vi "Glyph_MouseDown.vi"(6 "Double Click":bool, 8 "error in":errorcluster, 9 "Coords":T5, 10 "CtlRef":refnum<vi>, 11 "Data in":T1={"Class"={"Ants"=refnum, "Layer"=refnum, "Templates"=refnum, "Icon"=refnum, "Glyph"=refnum, "Settings"=refnum, "Tools"=refnum}, "Ref"={"Add Layer"=refnum, "Remove Layer"=refnum, "Line Text"=[], "Body Text Spec"=refnum, "DNL_Font"=refnum, "glyph path str"=refnum, "templates path str"=refnum, "Arrow Up"=refnum, "Arrow Down"=refnum, "IE VI Ref"=refnum, "Glyphs tree"=refnum, "Templates tree"=refnum, "Layer Icon Text"=refnum, "Layer Template"=refnum, "Body Text"=refnum, "Search Templates"=refnum, "TextMarker"=refnum, "Tab Control"=refnum, "Search Glyphs"=refnum, "Line Color"=refnum, "DNL_Glyphs []"=refnum, "Fill Color"=refnum, "Tools"=refnum, "Icon"=refnum, "Preview"=refnum, "Ants"=refnum, "Terminals"=refnum, "menu reference"=refnum, "LayerNames"=[], "GlyphLoadAnimation"=refnum, "TemplateLoadAnimation"=refnum, "refreshGlyphs"=refnum, "refreshTemplates"=refnum}, "Support"={"AntsRect"={"left"=0, "top"=0, "right"=0, "bottom"=0}, "Mouse Move Coords"={"Horizontal"=0, "Vertical"=0}, "Mouse Down Coords"={"Horizontal"=0, "Vertical"=0}, "Temp Coord"={"Horizontal"=0, "Vertical"=0}, "Action"=enum."Default", "Edge Color"=4914962, "Fill Color"=16860, "Mouse Down?"=FALSE, "Draft Mode?"=FALSE, "Temp Icon"=bytes[3102], "CTRL Pressed"=FALSE, "Move Selection?"=FALSE, "AntsRect Orig"={"left"=0, "top"=0, "right"=0, "bottom"=0}, "Text"="", "TM Set?"=FALSE, "Mouse inside icon?"=FALSE, "Tool (old value)"=0, "Pencil Move Color"=0, "Swap Colors?"=FALSE, "Shift pressed?"=FALSE}}) -> (0 "error out":errorcluster, 3 "Data out":T1={"Class"={"Ants"=refnum, "Layer"=refnum, "Templates"=refnum, "Icon"=refnum, "Glyph"=refnum, "Settings"=refnum, "Tools"=refnum}, "Ref"={"Add Layer"=refnum, "Remove Layer"=refnum, "Line Text"=[], "Body Text Spec"=refnum, "DNL_Font"=refnum, "glyph path str"=refnum, "templates path str"=refnum, "Arrow Up"=refnum, "Arrow Down"=refnum, "IE VI Ref"=refnum, "Glyphs tree"=refnum, "Templates tree"=refnum, "Layer Icon Text"=refnum, "Layer Template"=refnum, "Body Text"=refnum, "Search Templates"=refnum, "TextMarker"=refnum, "Tab Control"=refnum, "Search Glyphs"=refnum, "Line Color"=refnum, "DNL_Glyphs []"=refnum, "Fill Color"=refnum, "Tools"=refnum, "Icon"=refnum, "Preview"=refnum, "Ants"=refnum, "Terminals"=refnum, "menu reference"=refnum, "LayerNames"=[], "GlyphLoadAnimation"=refnum, "TemplateLoadAnimation"=refnum, "refreshGlyphs"=refnum, "refreshTemplates"=refnum}, "Support"={"AntsRect"={"left"=0, "top"=0, "right"=0, "bottom"=0}, "Mouse Move Coords"={"Horizontal"=0, "Vertical"=0}, "Mouse Down Coords"={"Horizontal"=0, "Vertical"=0}, "Temp Coord"={"Horizontal"=0, "Vertical"=0}, "Action"=enum."Default", "Edge Color"=4914962, "Fill Color"=16860, "Mouse Down?"=FALSE, "Draft Mode?"=FALSE, "Temp Icon"=bytes[3102], "CTRL Pressed"=FALSE, "Move Selection?"=FALSE, "AntsRect Orig"={"left"=0, "top"=0, "right"=0, "bottom"=0}, "Text"="", "TM Set?"=FALSE, "Mouse inside icon?"=FALSE, "Tool (old value)"=0, "Pencil Move Color"=0, "Swap Colors?"=FALSE, "Shift pressed?"=FALSE}})   [LabVIEW 2025]
doc: "Performs the actions necessary when there is a Mouse Down event on the Glyph array."
uses:
  <vilib>/Utility/miscctls.llb/LVPoint32TypeDef.ctl
  <resource>/plugins/NIIconEditor/Controls/Global Data.ctl
  <resource>/plugins/NIIconEditor/Class/Ants/Ants.lvclass
  <resource>/plugins/NIIconEditor/Class/FakedArray/FakedArray.lvclass
  <vilib>/LabVIEW Icon API/lv_icon/Classes/Icon/Icon.lvclass
  <resource>/plugins/NIIconEditor/Class/Icon Library/Glyph.lvclass
  <resource>/plugins/NIIconEditor/Class/Settings/Settings.lvclass
  <resource>/plugins/NIIconEditor/Class/Tools/Tools Paint.lvclass
  <resource>/plugins/NIIconEditor/Controls/IE Classes.ctl
  <resource>/plugins/NIIconEditor/Controls/References Cluster.ctl
  <resource>/plugins/NIIconEditor/Controls/SupportClass.ctl
  <resource>/plugins/NIIconEditor/Controls/SupportClass_Action.ctl
  <vilib>/LabVIEW Icon API/lv_icon/Controls/IEColor.ctl
  <vilib>/LabVIEW Icon API/lv_icon/Controls/Graphic.ctl
  <resource>/plugins/NIIconEditor/Controls/Tools.ctl
  <vilib>/LabVIEW Icon API/lv_icon/lv_icon.lvlib
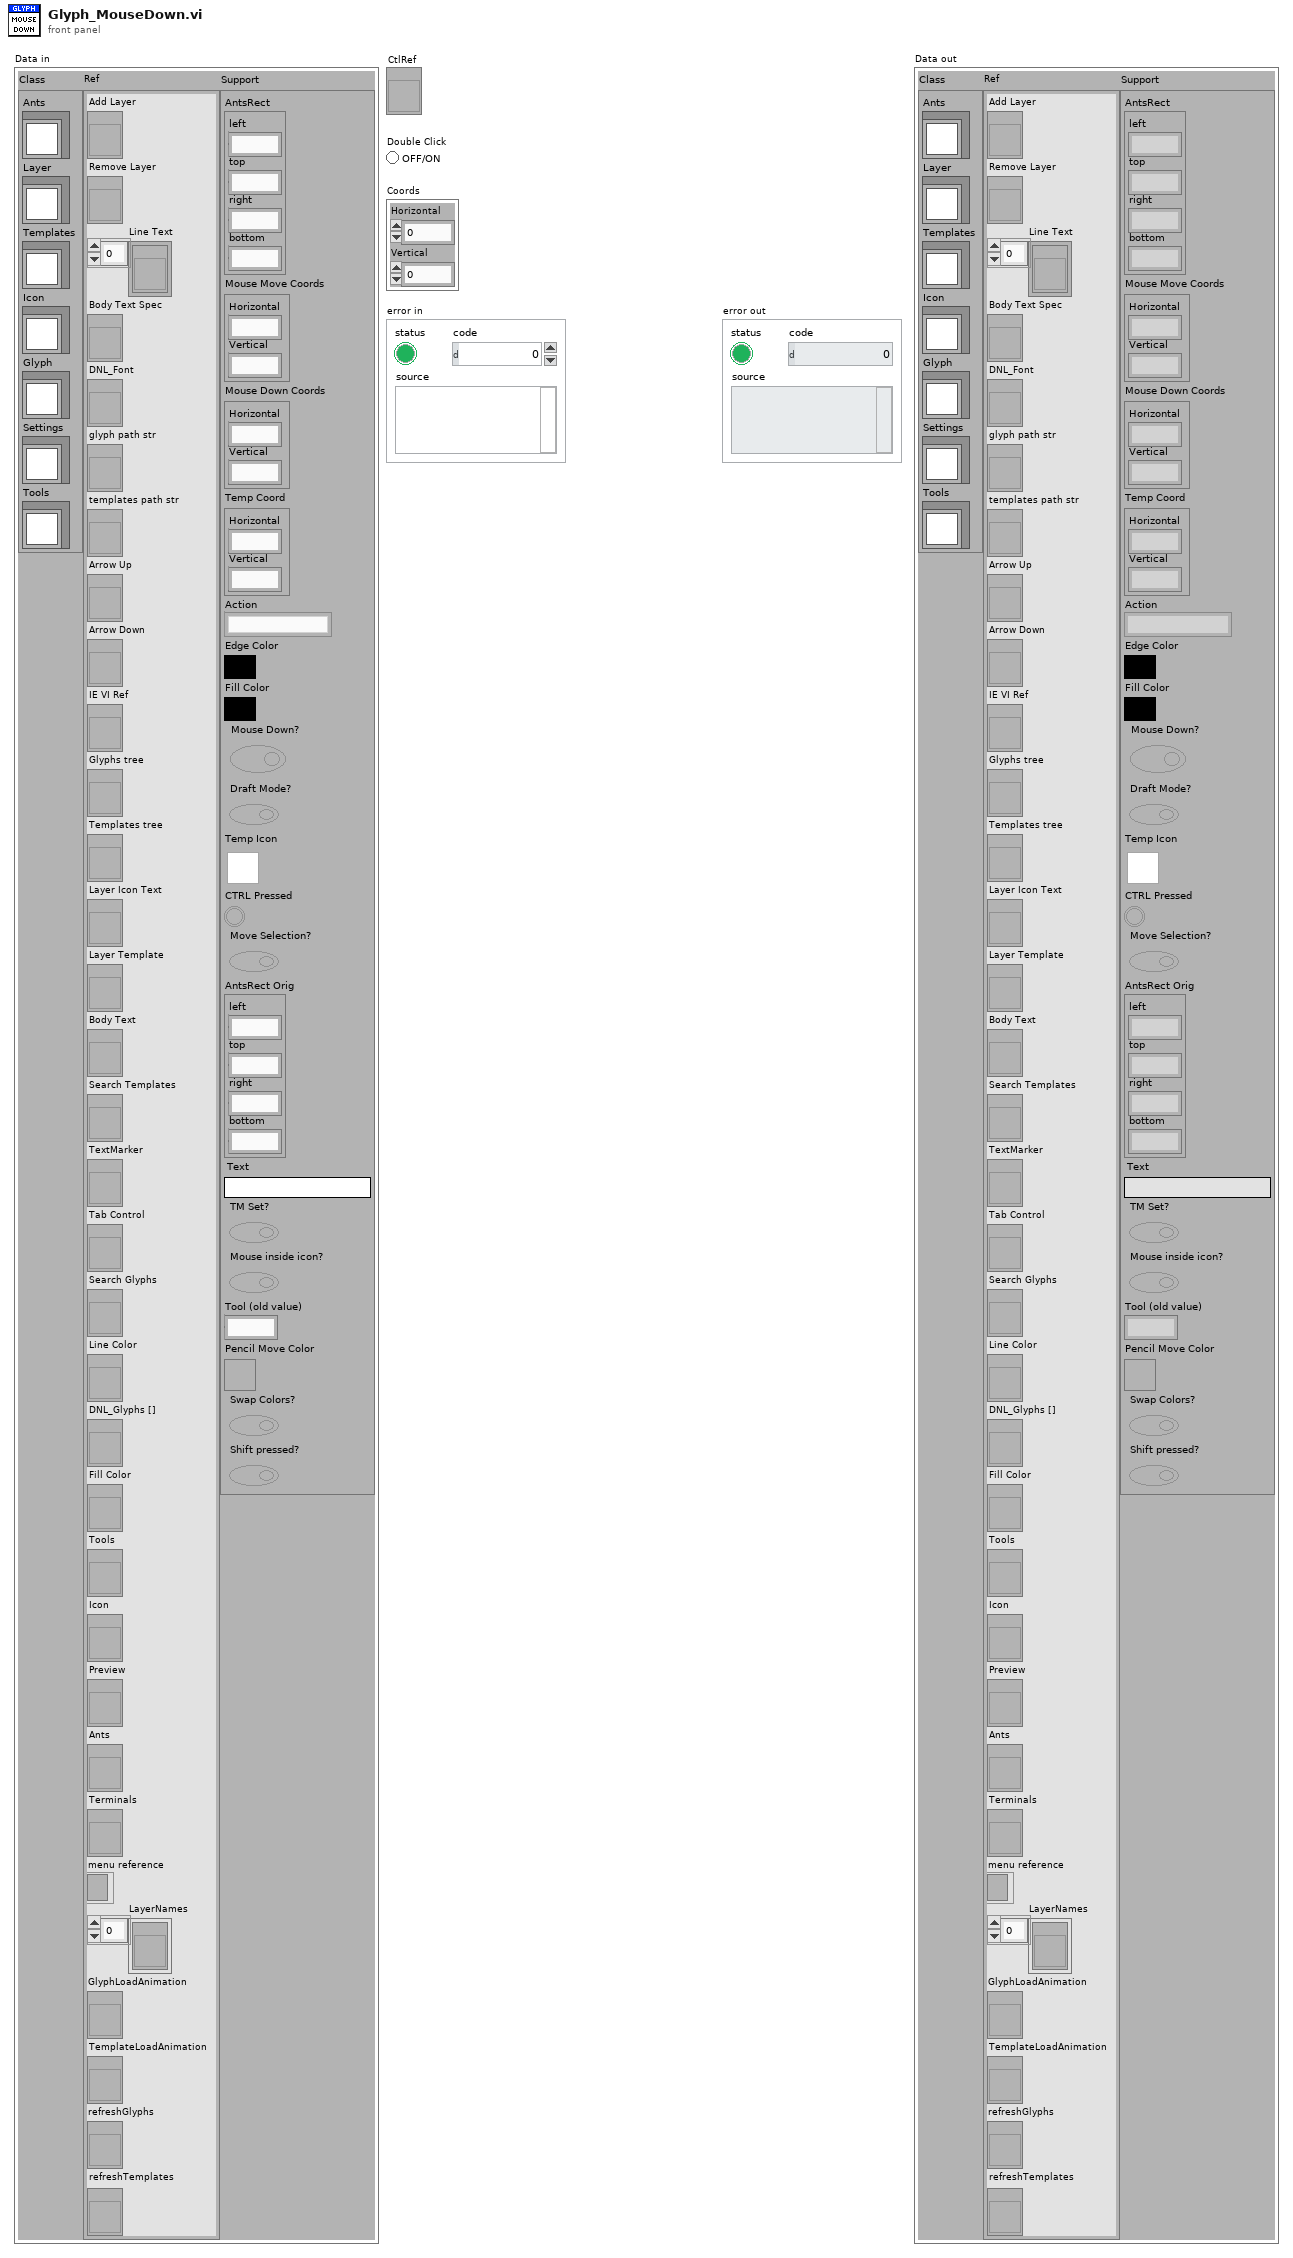
[diagram p1: front panel]
types:
  T1 = typedef "lv_icon.lvlib/Global Data.ctl" = cluster{"Class":T2, "Ref":T3, "Support":T4}
  T2 = typedef "IE Classes.ctl" = cluster{"Ants":refnum<class "Ants.lvclass">, "Layer":refnum<class "FakedArray.lvclass">, "Templates":refnum<class "FakedArray.lvclass">, "Icon":refnum<class "Icon.lvclass">, "Glyph":refnum<class "Glyph.lvclass">, "Settings":refnum<class "Settings.lvclass">, "Tools":refnum<class "Tools Paint.lvclass">}
  T3 = typedef "lv_icon.lvlib/References Cluster.ctl" = cluster{"Add Layer":refnum<vi>, "Remove Layer":refnum<vi>, "Line Text":refnum<vi>[], "Body Text Spec":refnum<vi>, "DNL_Font":refnum<vi>, "glyph path str":refnum<vi>, "templates path str":refnum<vi>, "Arrow Up":refnum<vi>, "Arrow Down":refnum<vi>, "IE VI Ref":refnum<vi>, "Glyphs tree":refnum<vi>, "Templates tree":refnum<vi>, "Layer Icon Text":refnum<vi>, "Layer Template":refnum<vi>, "Body Text":refnum<vi>, "Search Templates":refnum<vi>, "TextMarker":refnum<vi>, "Tab Control":refnum<vi>, "Search Glyphs":refnum<vi>, "Line Color":refnum<vi>, "DNL_Glyphs []":refnum<vi>, "Fill Color":refnum<vi>, "Tools":refnum<vi>, "Icon":refnum<vi>, "Preview":refnum<vi>, "Ants":refnum<vi>, "Terminals":refnum<vi>, "menu reference":refnum<k9>, "LayerNames":refnum<vi>[], "GlyphLoadAnimation":refnum<vi>, "TemplateLoadAnimation":refnum<vi>, "refreshGlyphs":refnum<vi>, "refreshTemplates":refnum<vi>}
  T4 = typedef "SupportClass.ctl" = cluster{"AntsRect":cluster{"left":i16, "top":i16, "right":i16, "bottom":i16}, "Mouse Move Coords":T5, "Mouse Down Coords":T5, "Temp Coord":T5, "Action":T6, "Edge Color":T7, "Fill Color":T7, "Mouse Down?":bool, "Draft Mode?":bool, "Temp Icon":picture, "CTRL Pressed":bool, "Move Selection?":bool, "AntsRect Orig":cluster{"left":i16, "top":i16, "right":i16, "bottom":i16}, "Text":string, "TM Set?":bool, "Mouse inside icon?":bool, "Tool (old value)":u32, "Pencil Move Color":u32, "Swap Colors?":bool, "Shift pressed?":bool}
  T5 = typedef "LVPoint32TypeDef.ctl" = cluster{"Horizontal":i32, "Vertical":i32}
  T6 = typedef "SupportClass_Action.ctl" = enum16{"Default", "Move Selection", "Glyph Library", "Tool"}
  T7 = typedef "IEColor.ctl" = u32
  T8 = typedef "Graphic.ctl" = cluster{"Rectangle":cluster{"left":i16, "top":i16, "right":i16, "bottom":i16}, "Path":path, "Image":picture, "Filter":string, "FileName":string}
  T9 = typedef "Tools.ctl" = enum32{"Pencil", "Line", "Dropper", "Fill", "Rectangle", "Filled Rectangle", "Ellipse", "Filled Ellipse", "Eraser", "Text", "Select", "Move"}
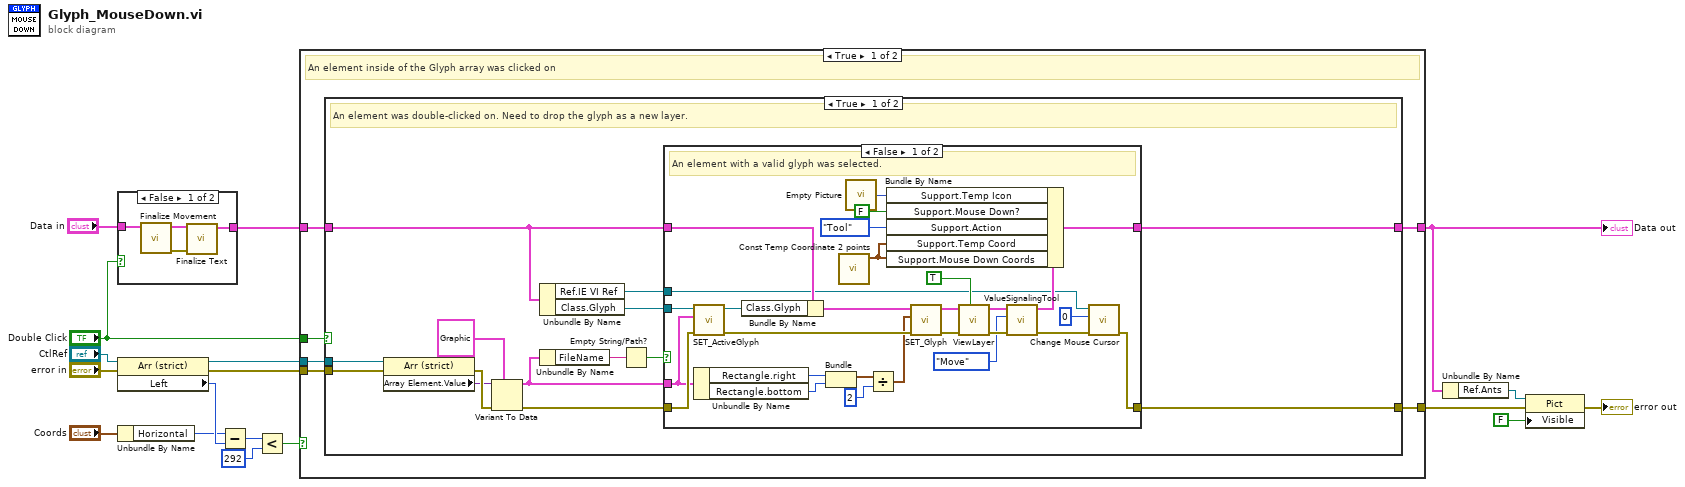
[diagram p0: block diagram]
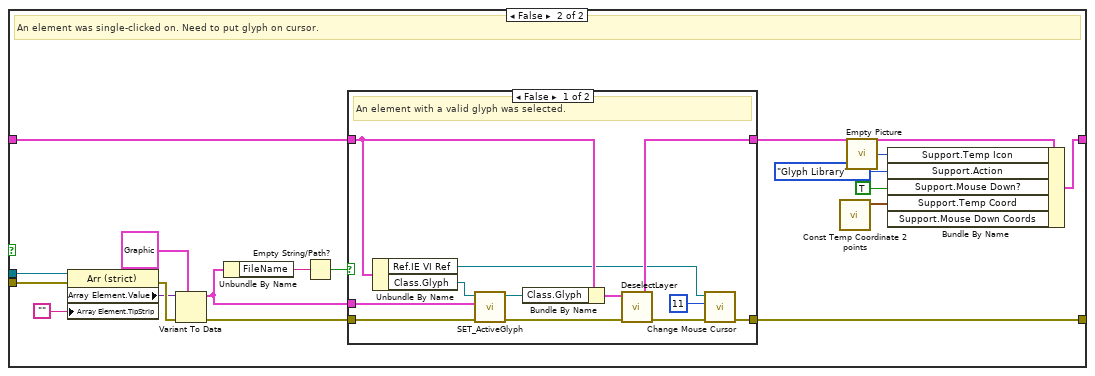
[diagram p4: hidden frame]
diagram:
  n1 = case shown="False" "Double Click" {
    tunnel: "Data in" -> [w21 w23]
    tunnel: [w19 w23] -> w6
    frame False {
      n2 = call <resource>:"Finalize Movement.vi"("Data in"=w21) -> ("error out"=w22:errorcluster, "Data out"=w20:T1)  [unwired: 2 in, 7 out]
      n3 = call <resource>:"Finalize Text.vi"("error in (no error)"=w22, "Data in"=w20) -> ("Data out"=w19:T1)  [unwired: 9 out]
    }
    frame True {
    }
  }
  n4 = property class="Arr (strict)"(reference="CtlRef", error in="error in") -> (reference out=w4:refnum<vi>, error out=w15:errorcluster, "Left"=w2:i32)
  n5 = Unbundle By Name("Coords") -> ("Horizontal"=w1:i32)
  n6 = Subtract(x=w1, y=w2) -> (x-y=w3:i32)
  n7 = Less?(x=w3, y=292 ("x")) -> (x < y?=w9:bool)
  n8 = case shown="True" w9 {
    tunnel: w4 -> [w27 _]
    tunnel: w15 -> [w29 w107]
    tunnel: [w28 w107] -> w18
    tunnel: "Double Click" -> [w26 _]
    tunnel: w6 -> [w25 w106]
    tunnel: [w24 w106] -> w5
    frame True {
      # "An element inside of the Glyph array was clicked on"
      n9 = case shown="True" w26 {
        tunnel: w27 -> [w39 w87]
        tunnel: w29 -> [w41 w90]
        tunnel: [w40 w89] -> w28
        tunnel: w25 -> [w35 w79]
        tunnel: [w34 w77] -> w24
        frame True {
          # "An element was double-clicked on. Need to drop the glyph as a new layer."
          n10 = property class="Arr (strict)"(reference=w39, error in=w41) -> (error out=w43:errorcluster, "Array Element.Value"=w38:variant)  [unwired: 1 out]
          n11 = Variant To Data(error in=w43, type=T8 {"Rectangle"={"left"=0, "top"=0, "right"=0, "bottom"=0}, "Path"=path "", "Image"=bytes[0], "Filter"="", "FileName"=""} ("Path & Icon"), Variant=w38) -> (data=w31:T8, error out=w42:errorcluster)
          n12 = Unbundle By Name(w35) -> ("Ref.IE VI Ref"=w33:refnum<vi>, "Class.Glyph"=w36:refnum<class "Glyph.lvclass">)
          n13 = Unbundle By Name(w31) -> ("FileName"=w32:string)
          n14 = Empty String/Path?(string/path=w32) -> (empty?=w30:bool)
          n15 = case shown="False" w30 {
            tunnel: w42 -> [w71 w73]
            tunnel: w36 -> [w55 _]
            tunnel: w35 -> [w53 w72]
            tunnel: [w52 w72] -> w34
            tunnel: w33 -> [w45 _]
            tunnel: [w66 w73] -> w40
            tunnel: w31 -> [w44 _]
            frame False {
              # "An element with a valid glyph was selected."
              n16 = call-dynamic "SET_ActiveGlyph.vi"("error in (no error)"=w71, "Active Glyph"=w44, "Glyph in"=w55) -> ("error out"=w68:errorcluster, "Glyph out"=w54:refnum<class "Glyph.lvclass">)  [unwired: 7 out]
              n17 = Unbundle By Name(w44) -> ("Rectangle.right"=w65:i16, "Rectangle.bottom"=w64:i16)
              n18 = Bundle By Name(cluster=w53, "Class.Glyph"=w54) -> (w51:T1)
              n19 = Bundle("right"=w65, "bottom"=w64) -> (w63:cluster{"right":i16, "bottom":i16})  [unwired: 1 out]
              n20 = call <resource>:"Const Temp Coordinate 2 points.vi"() -> ("Const Temp Coordinate"=w57:T5)  [unwired: 11 out]
              n21 = call "Empty Picture"() -> ("empty picture"=w58:picture)
              n22 = Divide(x=w63, y=2) -> (x/y=w61:cluster{"right":dbl, "bottom":dbl})
              n23 = call <resource>:"SET_Glyph.vi"("error in"=w68, "Coordinates"=w61, "Data in"=w51) -> ("error out"=w70:errorcluster, "Data out"=w50:T1)  [unwired: 7 out]
              n24 = call <resource>:"ViewLayer.vi"("Add to Undo?"=TRUE, "error in (no error)"=w70, "Data in"=w50) -> ("error out"=w69:errorcluster, "Data out"=w48:T1)  [unwired: 2 in, 5 out]
              n25 = call <resource>:"ValueSignalingTool.vi"("error in (no error)"=w69, "Tools"=Tools."Move", "Data in"=w48) -> ("error out"=w67:errorcluster, "Data out"=w47:T1)  [unwired: 7 out]
              n26 = Bundle By Name(cluster=w47, "Support.Temp Icon"=w58, "Support.Mouse Down?"=FALSE ("Mouse Down?"), "Support.Action"=SupportClass_Action."Tool" ("Action"), "Support.Temp Coord"=w57, "Support.Mouse Down Coords"=w57) -> (w52:T1)
              n27 = call <resource>:"Change Mouse Cursor.vi"("error in (no error)"=w67, "icon"=u16 0, "VI reference (current VI)"=w45) -> ("error out"=w66:errorcluster)  [unwired: 8 out]
            }
            frame True {
            }
          }
        }
        frame False {
          # "An element was single-clicked on. Need to put glyph on cursor."
          n28 = property class="Arr (strict)"(reference=w87, error in=w90, "Array Element.TipStrip"="") -> (error out=w91:errorcluster, "Array Element.Value"=w86:variant)  [unwired: 1 out]
          n29 = Variant To Data(error in=w91, type=T8 {"Rectangle"={"left"=0, "top"=0, "right"=0, "bottom"=0}, "Path"=path "", "Image"=bytes[0], "Filter"="", "FileName"=""} ("Path & Icon 2"), Variant=w86) -> (data=w76:T8, error out=w88:errorcluster)
          n30 = Unbundle By Name(w76) -> ("FileName"=w74:string)
          n31 = Empty String/Path?(string/path=w74) -> (empty?=w75:bool)
          n32 = case shown="False" w75 {
            tunnel: [w102 w105] -> w89
            tunnel: w88 -> [w101 w105]
            tunnel: w79 -> [w98 w104]
            tunnel: [w94 w104] -> w78
            tunnel: w76 -> [w93 _]
            frame False {
              # "An element with a valid glyph was selected."
              n33 = Unbundle By Name(w98) -> ("Ref.IE VI Ref"=w92:refnum<vi>, "Class.Glyph"=w96:refnum<class "Glyph.lvclass">)
              n34 = call-dynamic "SET_ActiveGlyph.vi"("error in (no error)"=w101, "Active Glyph"=w93, "Glyph in"=w96) -> ("error out"=w100:errorcluster, "Glyph out"=w97:refnum<class "Glyph.lvclass">)  [unwired: 7 out]
              n35 = Bundle By Name(cluster=w98, "Class.Glyph"=w97) -> (w95:T1)
              n36 = call <resource>:"DeselectLayer.vi"("error in (no error)"=w100, "Data in"=w95) -> ("error out"=w103:errorcluster, "Data out"=w94:T1)  [unwired: 8 out]
              n37 = call <resource>:"Change Mouse Cursor.vi"("error in (no error)"=w103, "icon"=u16 11, "VI reference (current VI)"=w92) -> ("error out"=w102:errorcluster)  [unwired: 8 out]
            }
            frame True {
              # "An invalid glyph was selected."
            }
          }
          n38 = call <resource>:"Const Temp Coordinate 2 points.vi"() -> ("Const Temp Coordinate"=w81:T5)  [unwired: 11 out]
          n39 = call "Empty Picture"() -> ("empty picture"=w82:picture)
          n40 = Bundle By Name(cluster=w78, "Support.Temp Icon"=w82, "Support.Action"=SupportClass_Action."Glyph Library" ("Action"), "Support.Mouse Down?"=TRUE ("Mouse Down?"), "Support.Temp Coord"=w81, "Support.Mouse Down Coords"=w81) -> (w77:T1)
        }
      }
    }
    frame False {
      # "The scrollbar was clicked on"
    }
  }
  "Data out" <- w5
  n41 = Unbundle By Name(w5) -> ("Ref.Ants"=w10:refnum<vi>)
  n42 = property class="Pict"(reference=w10, error in=w18, "Visible"=FALSE) -> (error out=→"error out":errorcluster)  [unwired: 1 out]
